vi "Set Voltage Mode.vi"(8 "error in (no error)":errorcluster, 10 "Voltage Mode":T1, 11 "VISA resource name":refnum<visa-resource-name>) -> (0 "error out":errorcluster, 3 "VISA resource name out":refnum<visa-resource-name>)   [LabVIEW 2016, in "SR7270 Drivers.lvclass"]
uses:
  SR7270 Drivers.lvclass
  Typedefs/VMODE--enum.ctl
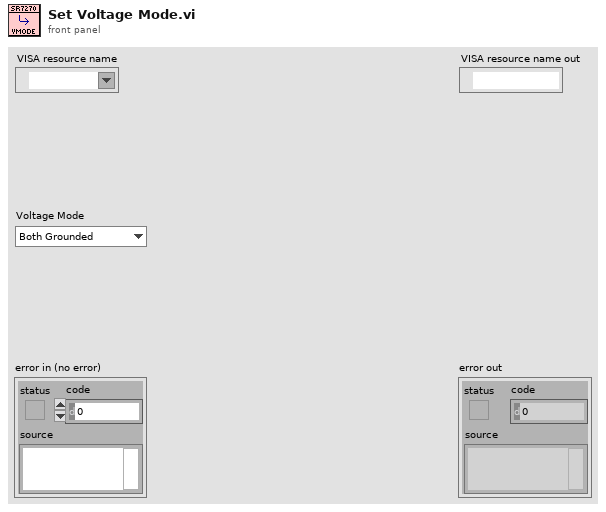
[diagram p1: front panel]
types:
  T1 = typedef "SR7270 Drivers.lvclass/VMODE--enum.ctl" = enum16{"Both Grounded", "A input only", "-B input only", "A-B differential"}
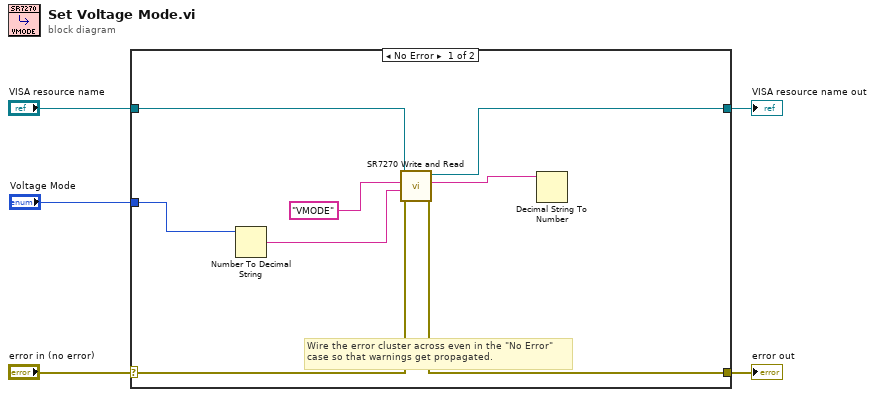
[diagram p0: block diagram]
diagram:
  n1 = case shown="No Error" "error in (no error)" {
    selector: "error in (no error)" -> [w13 w15]
    tunnel: [w12 w15] -> w4
    tunnel: [w6 w14] -> w2
    tunnel: "VISA resource name" -> [w7 w14]
    tunnel: "Voltage Mode" -> [w9 _]
    frame No Error {
      # "Wire the error cluster across even in the \"No Error\"\ncase so that warnings get propagated."
      n2 = Number To Decimal String(number=w9) -> (decimal integer string=w8:string)  [unwired: 1 in]
      n3 = call "SR7270 Write and Read.vi"("error in (no error)"=w13, "Parameter(s)"=w8, "Command Name"="VMODE", "VISA resource name"=w7) -> ("error out"=w12:errorcluster, "Read"=w10:string, "VISA resource name out"=w6:refnum<visa-resource-name>)  [unwired: 4 in, 1 out]
      n4 = Decimal String To Number(string=w10) -> ()  [unwired: 2 in, 2 out]
    }
    frame Error {
    }
  }
  "error out" <- w4
  "VISA resource name out" <- w2
